vi "Init (Section).vi"(6 "Index [-1, last]":i32=-1, 8 "error in (no error)":errorcluster, 10 "Name":string) -> (0 "error out":errorcluster, 3 "Find First Query out":refnum<class "Insert Query.lvclass">)   [LabVIEW 2013, in "Insert Query.lvclass"]
doc: "Copyright 2018, Carya Automatisering, Wiebe Walstra."
uses:
  Insert Query.lvclass
  Data.ctl
  Insert Query.lvclass/Insert Query.ctl
  CConfig Object.lvclass
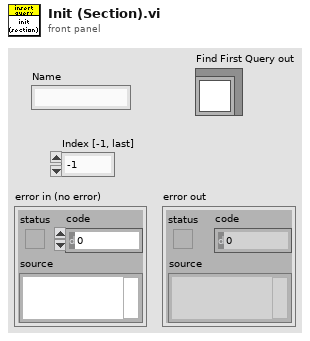
[diagram p1: front panel]
types:
  T1 = typedef "CConfig Object.lvclass/Data.ctl" = enum16{"pre", "name", "middle", "value", "post", "newline", "persistant", "tagged", "type"}
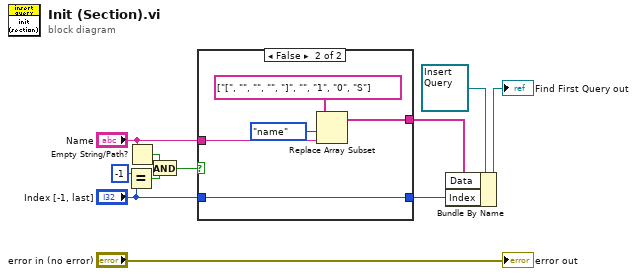
[diagram p0: block diagram]
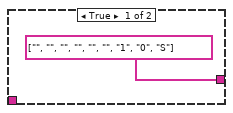
[diagram p2: hidden frame]
diagram:
  n1 = Equal?(x=-1, y="Index [-1, last]") -> (x = y?=w4:bool)
  n2 = Empty String/Path?(string/path="Name") -> (empty?=w5:bool)
  n3 = And(x=w5, y=w4) -> (x .and. y?=w1:bool)
  n4 = case shown="False" w1 {
    tunnel: "Name" -> [_ w17]
    tunnel: [string[] ["", "", "", "", "", "", "1", "0", "S"] ("Data") w16] -> w8
    tunnel: [_ w13] -> w3
    tunnel: "Index [-1, last]" -> [_ w13]
    frame True {
    }
    frame False {
      n5 = Replace Array Subset(array=string[] ["[", "", "", "", "]", "", "1", "0", "S"] ("Data"), new element=w17, index=Data."name" ("Data")) -> (w16:string[])
    }
  }
  n6 = Bundle By Name(cluster=refnum<class "Insert Query.lvclass"> refnum ("Find First Query in"), "Data"=w8, "Index"=w3) -> (→"Find First Query out":refnum<class "Insert Query.lvclass">)
  "error out" <- "error in (no error)"
